vi "Write Register.vi"(8 "error in (no error)":errorcluster, 9 "Value":u8 format="%x", 10 "Register":u8 format="%.0x", 11 "VISA resource name":refnum<visa-resource-name>) -> (0 "error out":errorcluster, 3 "VISA resource name out":refnum<visa-resource-name>)   [LabVIEW 2013, in "HadCon.lvlib"]
doc: "Write register value."
uses:
  <instrlib>/HadCon/HadCon.lvlib
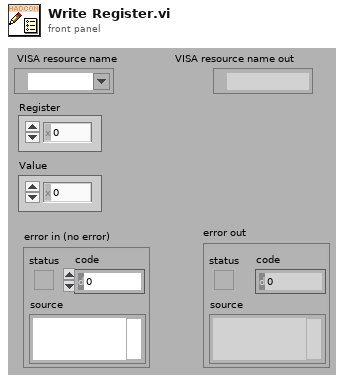
[diagram p1: front panel]
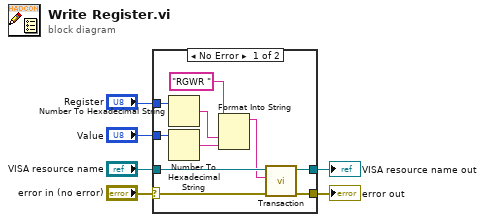
[diagram p0: block diagram]
diagram:
  n1 = case shown="No Error" "error in (no error)" {
    selector: "error in (no error)" -> [w10 w17]
    tunnel: [w8 w18] -> w6
    tunnel: "VISA resource name" -> [w11 w18]
    tunnel: [w7 w17] -> w4
    tunnel: "Register" -> [w14 _]
    tunnel: "Value" -> [w15 _]
    frame No Error {
      n2 = Number To Hexadecimal String(2:w14) -> (0:w13:string)  [unwired: 1 in]
      n3 = Number To Hexadecimal String(2:w15) -> (0:w12:string)  [unwired: 1 in]
      n4 = Format Into String(initial string="RGWR ", w13, w12) -> (resulting string=w9:string)  [unwired: 2 in, 1 out]
      n5 = call <instrlib>:"Transaction.vi"("Error In"=w10, "Command"=w9, "VISA resource name"=w11) -> ("Error Out"=w7:errorcluster, "VISA resource name out"=w8:refnum<visa-resource-name>)  [unwired: 6 in, 1 out]
    }
    frame Error {
    }
  }
  "VISA resource name out" <- w6
  "error out" <- w4
